vi "Pressure_Jog_Z.vi"() -> ()   [LabVIEW 2013]
uses:
  <vilib>/Analysis/baseanly.llb/Mean (DBL).vi
  <vilib>/LabVIEW Interface for Arduino/LabVIEW Interface for Arduino.lvlib
  <vilib>/Analysis/NI_AALBase.lvlib
panel:
  out "Current Z Position":sgl
  in  "MG17Motor":refnum<k7>(container)
  in  "Serial":i32=90848557
  out "Force Threshhold Reached":bool
  out "Force Average":dbl format="%0.2f"
  out "Force vs Time":dbl[](graph)
  out "Voltage Average":dbl format="%0.2f"
  in  "Array":dbl[](array[numeric])
  in  "Sample Rate (HZ)":u16
  in  "Analog Input Pin":u8
  in  "Stop":bool
  out "Volatege vs Time":dbl[](graph)
  out "output array":dbl[](array[numeric])
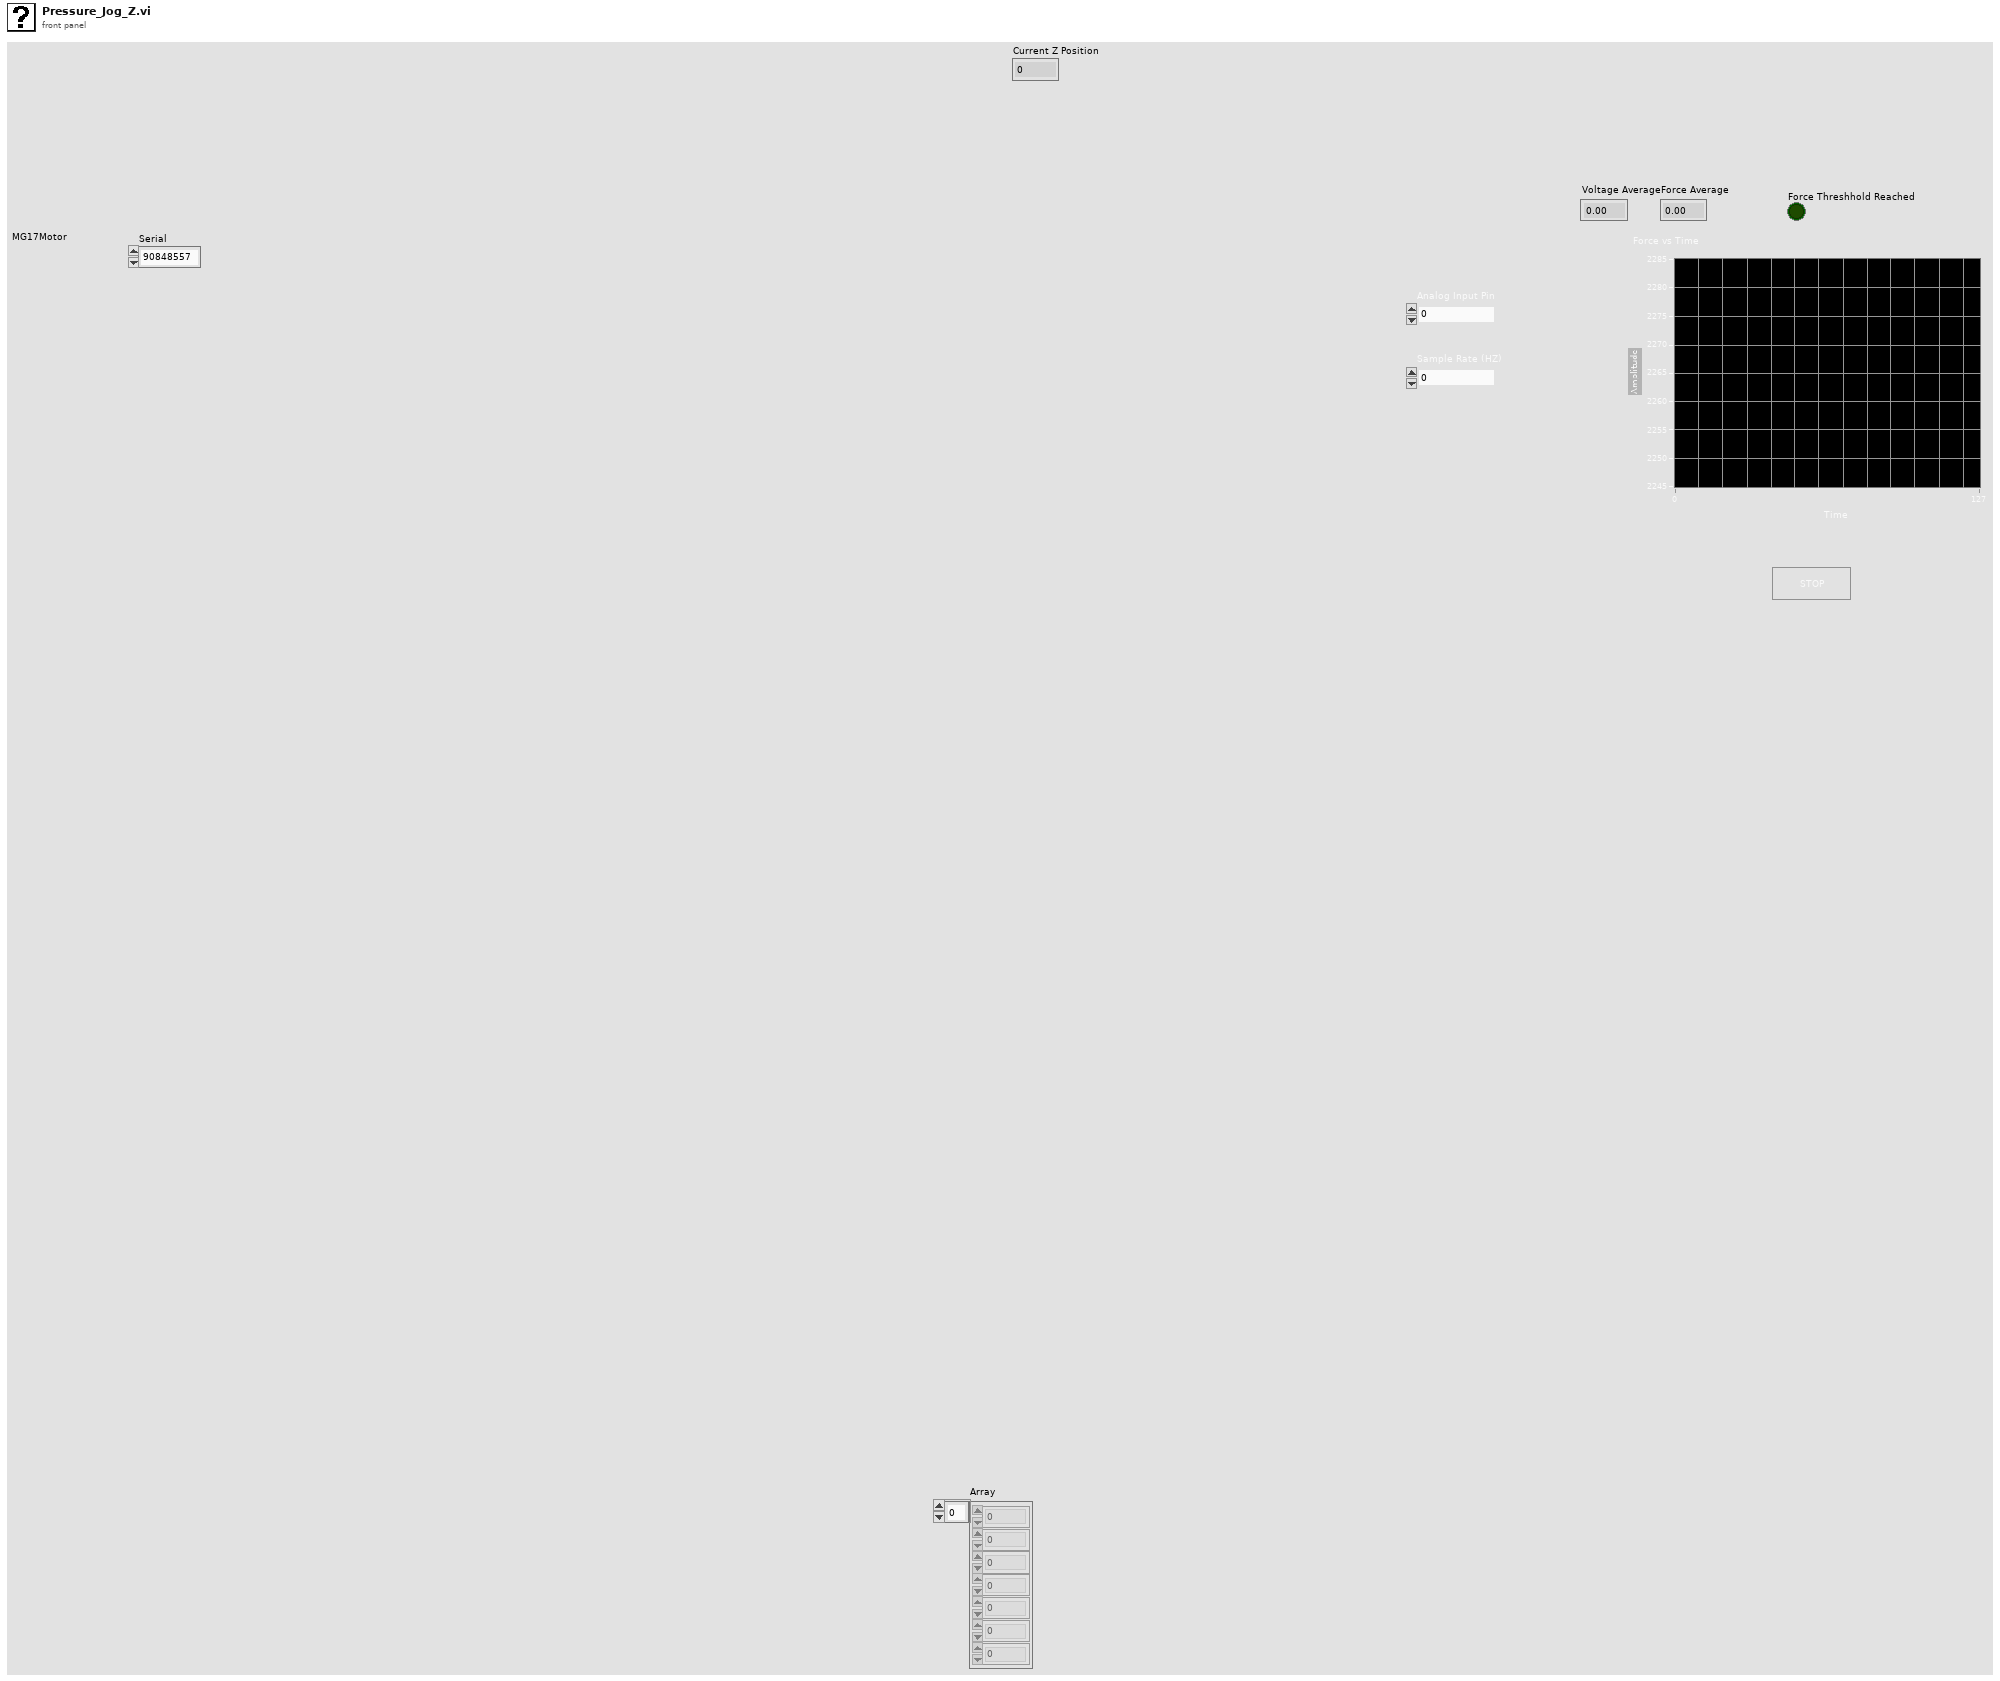
[diagram p1: front panel]
types:
  T1 = typedef "LabVIEW Interface for Arduino.lvlib/Arduino Resource.ctl" = cluster{"VISA resource":refnum<visa-resource-name>, "Board Type":T2, "Connection Type":enum8{"USB / Serial"}, "Bytes Per Packet (15)":u8}
  T2 = typedef "LabVIEW Interface for Arduino.lvlib/Board Type.ctl" = enum16{"Uno", "Dimuelanove w/Atmega 328", "Mega 2560"}
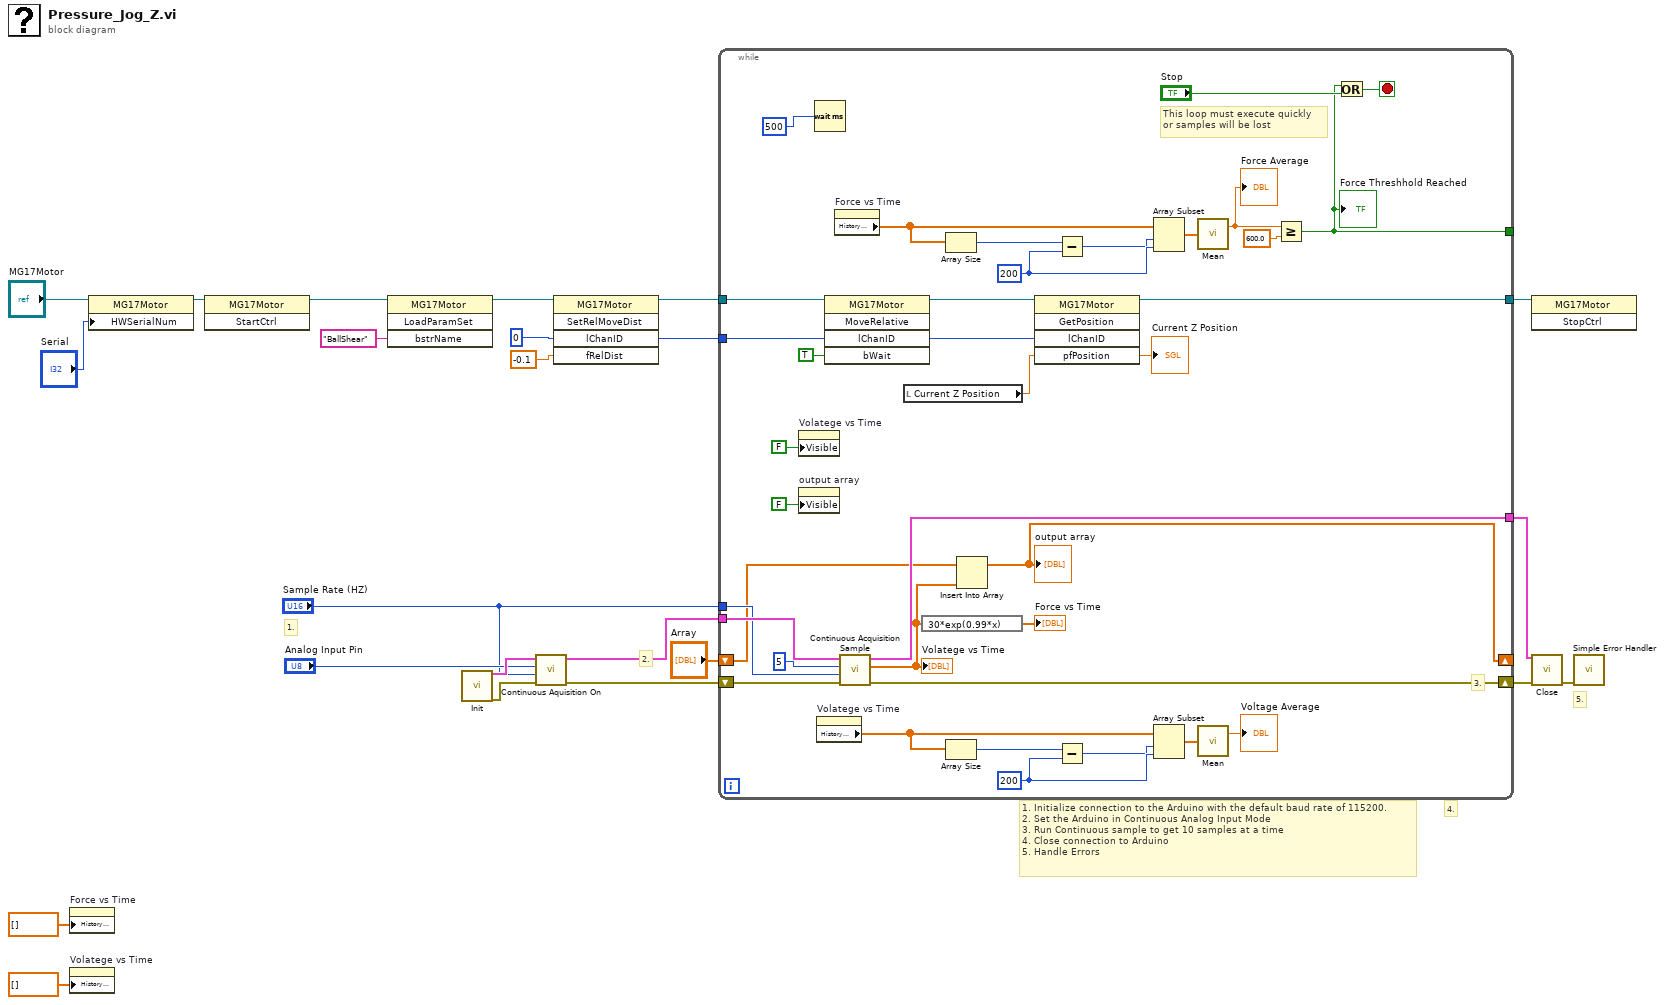
[diagram p0: block diagram]
diagram:
  # "5."
  # "4."
  # "2."
  # "1."
  # "1. Initialize connection to the Arduino with the default baud rate of 115200.\n2. Set the Arduino in Continuous Analog Input Mode\n3. Run Continuous sample to get 10 samples at a time\n4. Close connection to Arduino\n5. Handle Errors"
  n1 = property on="Force vs Time" class="WFChart (strict)"("History Data"=dbl[] []) -> ()  [unwired: 2 in, 2 out]
  n2 = property on="Volatege vs Time" class="WFChart (strict)"("History Data"=dbl[] []) -> ()  [unwired: 2 in, 2 out]
  n3 = property class="MG17Motor"(reference="MG17Motor", "HWSerialNum"="Serial") -> (reference out=w11:refnum<k7>)  [unwired: 1 in, 1 out]
  n4 = invoke class="MG17Motor" method="StartCtrl"(reference=w11) -> (reference out=w10:refnum<k7>)  [unwired: 2 in, 2 out]
  n5 = invoke class="MG17Motor" method="LoadParamSet"(reference=w10, "bstrName"="BallShear") -> (reference out=w6:refnum<k7>)  [unwired: 2 in, 3 out]
  n6 = call <vilib>:"Init.vi"() -> ("Arduino Resource"=w23:T1, "error out"=w16:errorcluster)  [unwired: 18 in]
  n7 = call <vilib>:"Continuous Aquisition On.vi"("error in"=w16, "Acquition Speed"="Sample Rate (HZ)", "Analog Input Pin"="Analog Input Pin", "Arduino Resource"=w23) -> ("error out"=w21:errorcluster, "Arduino Resource"=w22:T1)  [unwired: 6 in]
  n8 = invoke class="MG17Motor" method="SetRelMoveDist"(reference=w6, "lChanID"=0, "fRelDist"=-0.1) -> (reference out=w3:refnum<k7>, "lChanID"=w1:i32)  [unwired: 2 in, 3 out]
  n9 = while {
    tunnel: w22 -> [w60]
    tunnel: [w59] -> w20
    shift-right: [w58] -> w17
    shift-left: w21 -> [w57]
    tunnel: "Sample Rate (HZ)" -> [w55]
    shift-right: [w53] -> _
    shift-left: "Array" -> [w54]
    tunnel: [w33] -> _
    tunnel: w3 -> [w27]
    tunnel: [w26] -> w2
    tunnel: w1 -> [w25]
    stop <- w36 stop-if-true
    w44 = 200 ("length")
    w41 = 200 ("length")
    # "This loop must execute quickly\nor samples will be lost"
    # "3."
    n10 = property on="Volatege vs Time" class="WFChart (strict)"("Visible"=FALSE) -> ()  [unwired: 2 in, 2 out]
    n11 = property on="output array" class="Arr (strict)"("Visible"=FALSE) -> ()  [unwired: 2 in, 2 out]
    n12 = Wait (ms)(milliseconds to wait=500) -> ()  [unwired: 1 out]
    n13 = property on="Volatege vs Time" class="WFChart (strict)"() -> ("History Data"=w48:dbl[])  [unwired: 2 in, 2 out]
    n14 = invoke class="MG17Motor" method="MoveRelative"(reference=w27, "lChanID"=w25, "bWait"=TRUE) -> (reference out=w32:refnum<k7>, "lChanID"=w31:i32)  [unwired: 2 in, 3 out]
    n15 = property on="Force vs Time" class="WFChart (strict)"() -> ("History Data"=w50:dbl[])  [unwired: 2 in, 2 out]
    n16 = call <vilib>:"Continuous Acquisition Sample.vi"("Arduino Resource"=w60, "Samples to Read"=u16 5, "Sample Rate (HZ)"=w55, "error in (no error)"=w57) -> ("Arduino Resource"=w59:T1, "Data"=w52:dbl[], "error out"=w58:errorcluster)  [unwired: 4 in]
    "Volatege vs Time" <- w52
    n17 = local read "Current Z Position"() -> (w30:sgl)
    n18 = expression code="30*exp(0.99*x)"(w52) -> (→"Force vs Time":dbl[])
    n19 = Array Size(array=w50) -> (size(s)=w42:i32)
    n20 = Array Size(array=w48) -> (size(s)=w45:i32)
    n21 = Insert Into Array(array=w54, new element=w52) -> (w53:dbl[])  [unwired: 1 in]
    "output array" <- w53
    n22 = invoke class="MG17Motor" method="GetPosition"(reference=w32, "lChanID"=w31, "pfPosition"=w30) -> (reference out=w26:refnum<k7>, "pfPosition"=→"Current Z Position":sgl)  [unwired: 2 in, 3 out]
    n23 = Subtract(x=w42, y=w41) -> (x-y=w40:i32)
    n24 = Subtract(x=w45, y=w44) -> (x-y=w43:i32)
    n25 = Array Subset(array=w50, index=w40, length=w41) -> (w49:dbl[])
    n26 = Array Subset(array=w48, index=w43, length=w44) -> (w46:dbl[])
    n27 = call-poly <vilib>:"Mean.vi"("X"=w49) -> ("mean"=w39:dbl)  [unwired: 1 out]
    "Force Average" <- w39
    n28 = call-poly <vilib>:"Mean.vi"("X"=w46) -> ("mean"=→"Voltage Average":dbl)  [unwired: 1 out]
    n29 = Greater Or Equal?(x=w39, y=600.0) -> (x >= y?=w33:bool)
    "Force Threshhold Reached" <- w33
    n30 = Or(x=w33, y="Stop") -> (x .or. y?=w36:bool)
  }
  n31 = invoke class="MG17Motor" method="StopCtrl"(reference=w2) -> ()  [unwired: 2 in, 3 out]
  n32 = call <vilib>:"Close.vi"("Arduino Resource"=w20, "error in"=w17) -> ("error out"=w19:errorcluster)  [unwired: 13 in]
  n33 = call <vilib>:"Simple Error Handler.vi"("error in (no error)"=w19) -> ()  [unwired: 4 in, 5 out]
